vi "Plane Extraction and Mask.vi"(0 "error in":errorcluster) -> (1 "Image Out":T1(plugin-control), 2 "error out":errorcluster)   [LabVIEW 2009]
uses:
  <vilib>/vision/NI_Vision_Development_Module.lvlib
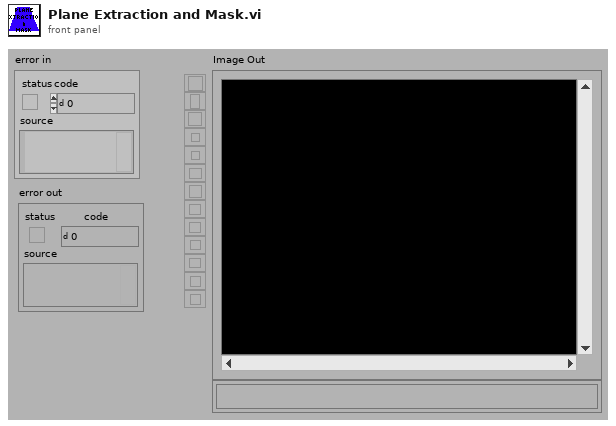
[diagram p1: front panel]
types:
  T1 = typedef "IMAQ Image.ctl" = refnum<image>
  T2 = cluster{"Global Rectangle":i32[], "Contours":cluster{"ID":enum32{"External", "Internal"}, "Type":u32, "Coordinates":i32[]}[]}
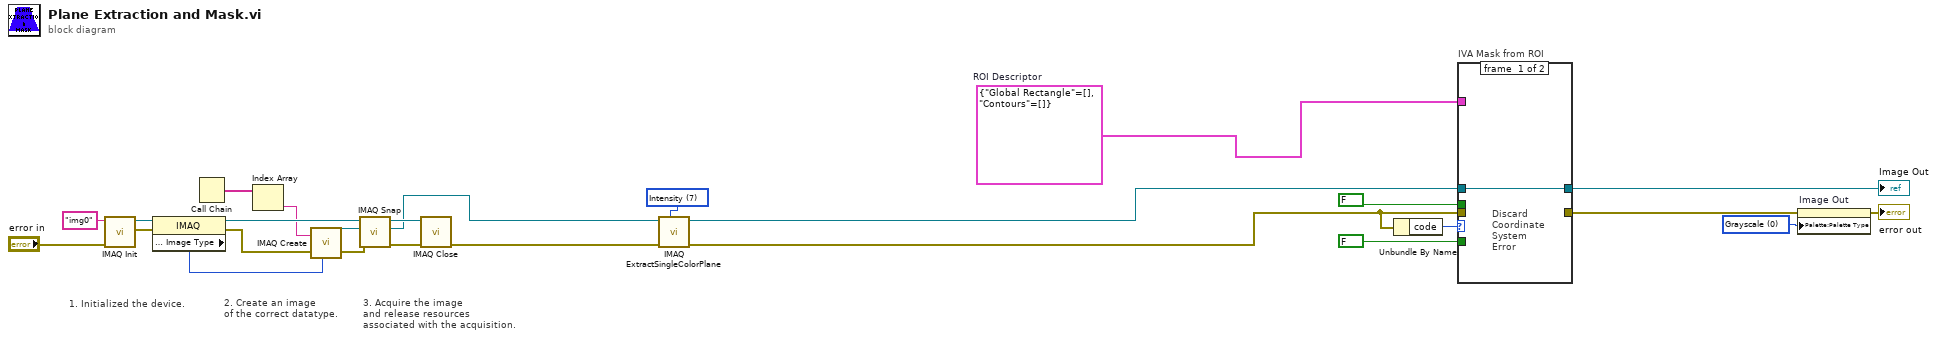
[diagram p0: block diagram]
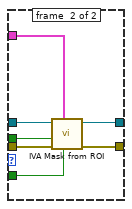
[diagram p2: hidden frame]
diagram:
  w2 = u32 0 items=["Grayscale", "Binary", "Gradient", "Rainbow", "Temperature", "User Defined"] ("Palette")
  w9 = T2 {"Global Rectangle"=[], "Contours"=[]}  # ROI Descriptor
  w12 = 7 items=["Red", "Green", "Blue", "Hue", "Saturation", "Luminance", "Value", "Intensity"] ("Color Plane")
  # "3. Acquire the image\nand release resources\nassociated with the acquisition."
  # "2. Create an image\nof the correct datatype."
  # "1. Initialized the device."
  n1 = call <vilib>:"IMAQ Init.vi"("error in (no error)"="error in", "Interface Name"="img0") -> ("error out"=w19:errorcluster, "IMAQ Session Out"=w20:refnum<k11>)  [unwired: 8 out]
  n2 = property class="IMAQ"(reference=w20, error in=w19) -> (reference out=w18:refnum<k11>, error out=w17:errorcluster, "Image Parameters : Image Type"=w26:u32)
  n3 = Call Chain() -> (call chain=w14:string[])
  n4 = Index Array(array=w14) -> (element=w13:string)  [unwired: 1 in]
  n5 = call "IMAQ Create"("Image Name"=w13, "Image Type"=w26, "error in (no error)"=w17) -> ("New Image"=w24:T1, "error out"=w16:errorcluster)  [unwired: 1 in, 1 out]
  n6 = call <vilib>:"IMAQ Snap.vi"("error in (no error)"=w16, "Image In"=w24, "IMAQ Session In"=w18) -> ("error out"=w22:errorcluster, "Image Out"=w11:T1, "IMAQ Session Out"=w23:refnum<k11>)  [unwired: 6 out]
  n7 = call <vilib>:"IMAQ Close.vi"("error in (no error)"=w22, "IMAQ Session In"=w23) -> ("error out"=w21:errorcluster)  [unwired: 9 out]
  n8 = call "IMAQ ExtractSingleColorPlane"("Color Plane"=w12, "error in (no error)"=w21, "Image Src"=w11) -> ("error out"=w10:errorcluster, "Image Dst Out"=w7:T1)  [unwired: 1 in, 6 out]
  n9 = Unbundle By Name(w10) -> ("code"=w4:i32)
  n10 = case "IVA Mask from ROI" shown="Default" w4 {
    tunnel: w9 -> [_ w34]
    tunnel: FALSE ("Shrink") -> [_ w33]
    tunnel: w7 -> [w27 w32]
    tunnel: w10 -> [_ w31]
    tunnel: [_ w30] -> w6
    tunnel: [w27 w29] -> w3
    tunnel: FALSE ("Out / In") -> [_ w28]
    frame #0 {
      # "Discard\nCoordinate\nSystem\nError"
    }
    frame #1 {
      n11 = call <vilib>:"IVA Mask from ROI.vi"("Shrink"=w33, "ROI Descriptor"=w34, "error in (no error)"=w31, "Out / In"=w28, "Image Src"=w32) -> ("error out"=w30:errorcluster, "Image Out"=w29:T1)  [unwired: 5 out]
    }
  }
  "Image Out" <- w3
  n12 = property on="Image Out" class="ImageControl"(error in=w6, "Palette:Palette Type"=w2) -> (error out=→"error out":errorcluster)  [unwired: 1 in, 1 out]
